vi "get_valve_state (SubVI).vi"(7 "error in":errorcluster, 10 "valve_monitors":tag="Dev3/ai0,Dev3/ai8") -> (0 "error out":errorcluster, 1 "valve_fault":bool, 2 "valve_closed":bool, 3 "valve_open":bool)   [LabVIEW 2022 SP3]
uses:
  <vilib>/DAQmx/read.llb/DAQmx Read (Analog 2D DBL NChan NSamp).vi
  <vilib>/Analysis/baseanly.llb/Mean (DBL).vi
  <vilib>/DAQmx/create/channels.llb/DAQmx Create Channel (AI-Voltage-Basic).vi
  <vilib>/DAQmx/configure/timing.llb/DAQmx Timing (Sample Clock).vi
  <vilib>/DAQmx/miscellaneous.llb/DAQmx Fill In Error Info.vi
  <vilib>/Analysis/NI_AALBase.lvlib
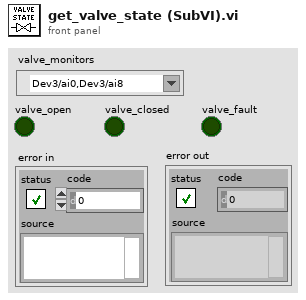
[diagram p1: front panel]
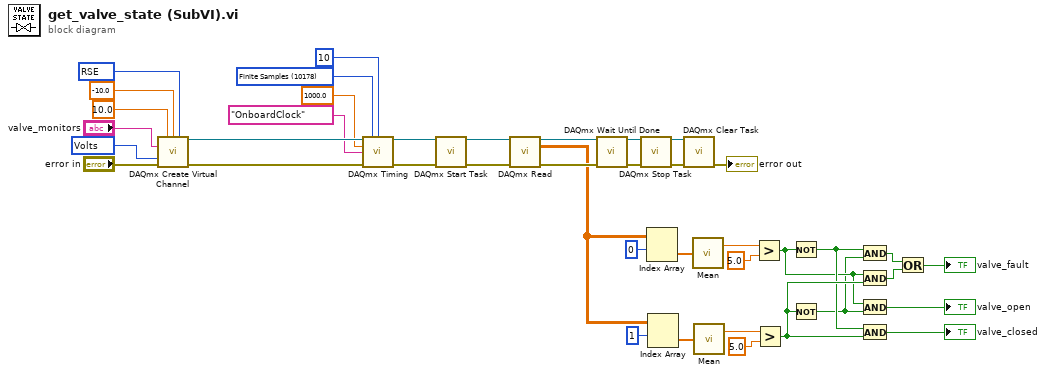
[diagram p0: block diagram]
diagram:
  w22 = 10178 items=["Finite Samples"=10178, "Continuous Samples"=10123, "Hardware Timed Single Point"=12522] ("sample mode")
  w37 = 10083 items=["default"=-1, "RSE"=10083, "NRSE"=10078, "Differential"=10106, "Pseudodifferential"=12529] ("input terminal configuration")
  w39 = 10348 items=["Volts"=10348, "From Custom Scale"=10065] ("units")
  n1 = call-poly <vilib>:"DAQmx Create Virtual Channel.vi"("maximum value"=10.0, "minimum value"=-10.0, "input terminal configuration"=w37, "physical channels"="valve_monitors", "units"=w39, "error in"="error in") -> ("task out"=w34:refnum<k21>, "error out"=w33:errorcluster)  [unwired: 8 in]
  n2 = call-poly <vilib>:"DAQmx Timing.vi"("task/channels in"=w34, "sample mode"=w22, "samples per channel"=10, "rate"=1000.0, "source"=tag "OnboardClock", "error in"=w33) -> ("task out"=w35:refnum<k21>, "error out"=w32:errorcluster)  [unwired: 8 in]
  n3 = call <vilib>:"DAQmx Start Task.vi"("task/channels in"=w35, "error in"=w32) -> ("task out"=w38:refnum<k21>, "error out"=w31:errorcluster)  [unwired: 12 in]
  n4 = call-poly <vilib>:"DAQmx Read.vi"("task/channels in"=w38, "error in"=w31) -> ("task out"=w23:refnum<k21>, "data"=w12:dbl[][], "error out"=w24:errorcluster)  [unwired: 11 in]
  n5 = call <vilib>:"DAQmx Wait Until Done.vi"("task/channels in"=w23, "error in"=w24) -> ("task out"=w28:refnum<k21>, "error out"=w27:errorcluster)  [unwired: 12 in]
  n6 = call <vilib>:"DAQmx Stop Task.vi"("task/channels in"=w28, "error in"=w27) -> ("task out"=w26:refnum<k21>, "error out"=w25:errorcluster)  [unwired: 12 in]
  n7 = Index Array(array=w12, index (row)=0) -> (element=w19:dbl[])  [unwired: 1 in]
  n8 = Index Array(array=w12, index (row)=1) -> (element=w15:dbl[])  [unwired: 1 in]
  n9 = call <vilib>:"DAQmx Clear Task.vi"("task in"=w26, "error in"=w25) -> ("error out"=→"error out":errorcluster)  [unwired: 13 in]
  n10 = call-poly <vilib>:"Mean.vi"("X"=w19) -> ("mean"=w18:dbl)  [unwired: 1 out]
  n11 = call-poly <vilib>:"Mean.vi"("X"=w15) -> ("mean"=w14:dbl)  [unwired: 1 out]
  n12 = Greater?(x=w18, y=5.0) -> (0:w9:bool)
  n13 = Greater?(x=w14, y=5.0) -> (0:w11:bool)
  n14 = Not(x=w9) -> (.not. x?=w10:bool)
  n15 = Not(x=w11) -> (.not. x?=w8:bool)
  n16 = And(x=w10, y=w8) -> (x .and. y?=w7:bool)
  n17 = And(x=w9, y=w11) -> (x .and. y?=w6:bool)
  n18 = And(x=w9, y=w8) -> (x .and. y?=→"valve_open":bool)
  n19 = And(x=w10, y=w11) -> (x .and. y?=→"valve_closed":bool)
  n20 = Or(x=w7, y=w6) -> (x .or. y?=→"valve_fault":bool)
